vi "Read Full Output.vi"(6 "maximal byte count (-1)":i32=-1, 7 "timeout [ms]":u32, 8 "error in":errorcluster, 11 "GOLPI ref. in":T1={"pipe handle"={"lv_proc.dll file path"=path "", "process instance handle"=[], "debug mode"=FALSE, "debug data"=[]}, "fast read timeout [ms]"=500, "fast read settle time [ms]"=10, "fast read to multiple [ms]"=1, "max elements per input line"=100, "slow read timeout [ms]"=5000, "stdin double format specifier"="%_16e", "max elements per stdout output column"=100}) -> (0 "error out":errorcluster, 2 "read buffer":string, 3 "GOLPI ref. out":T1={"pipe handle"={"lv_proc.dll file path"=path "", "process instance handle"=[], "debug mode"=FALSE, "debug data"=[]}, "fast read timeout [ms]"=500, "fast read settle time [ms]"=10, "fast read to multiple [ms]"=1, "max elements per input line"=100, "slow read timeout [ms]"=5000, "stdin double format specifier"="%_16e", "max elements per stdout output column"=100}, 5 "bytes remaining":i32)   [LabVIEW 2013, in "GOLPI library.lvlib"]
doc: "Reads full output of GNU Octave in stdout pipe.\nIf timeout is exceeded (i.e. buffer contains too many characters), returns only part of buffer and returns number of bytes remaining in the stdout (if any).\nReading also stops if maximal byte count terminal is set to natural nonzero value and number of red bytes reaches this limit."
uses:
  GOLPI library.lvlib
  Private/Type Definitions/GOLPI reference Type Def.ctl
  LV Process source distribution/Pipe Handle.ctl
  Private/Type Definitions/Custom Error Codes Enum Type Def.vi
  LV Process source distribution/LV Process library.lvlib
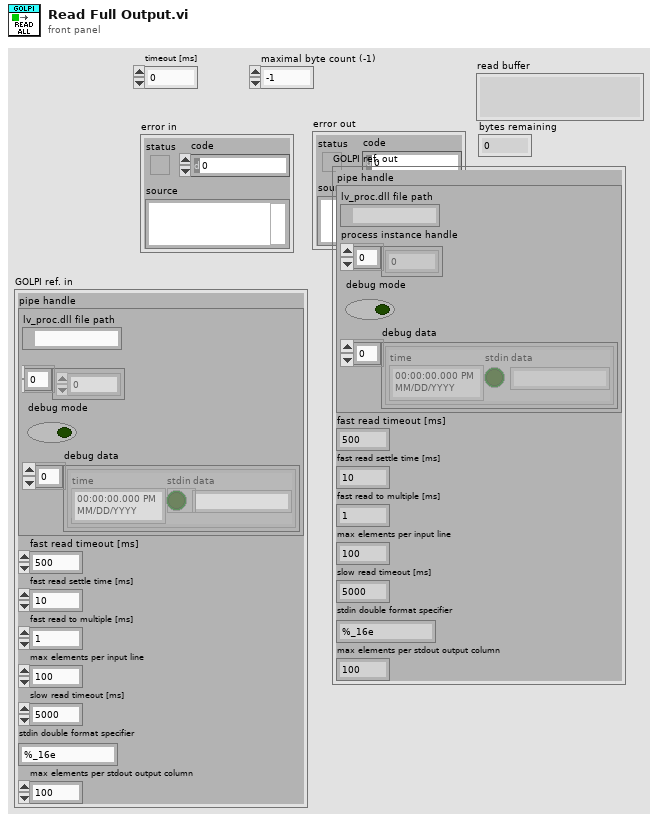
[diagram p1: front panel]
types:
  T1 = typedef "GOLPI library.lvlib/GOLPI reference Type Def.ctl" = cluster{"pipe handle":T2, "fast read timeout [ms]":u32, "fast read settle time [ms]":u32, "fast read to multiple [ms]":u32, "max elements per input line":u32, "slow read timeout [ms]":u32, "stdin double format specifier":string, "max elements per stdout output column":u32}
  T2 = typedef "LV Process library.lvlib/Pipe Handle.ctl" = cluster{"lv_proc.dll file path":path, "process instance handle":u32[], "debug mode":bool, "debug data":cluster{"time":timestamp, "stdin":bool, "data":string}[]}
  T3 = typedef "GOLPI library.lvlib/Custom Error Codes Enum Type Def.vi" = enum16{"no error", "00 working directory PAR1 missing", "01 octave binary PAR1 missing", "02 octave report error PAR1", "03 empty output last cmd PAR1", "04 missing temporary file PAR1", "05 pwd PAR 1 not exist", "10 var PAR1 not string, vect", "11 var PAR1 not num, scal, ~compl", "12 var PAR1 not num, scal, compl", "13 var PAR1 not num, vect, ~compl", "14 var PAR1 not num, vect, compl", "15 var PAR1 not num, mat, ~compl", "16 var PAR1 not num, mat, ~compl", "30 WARNING read timeout", "99 not finished"}
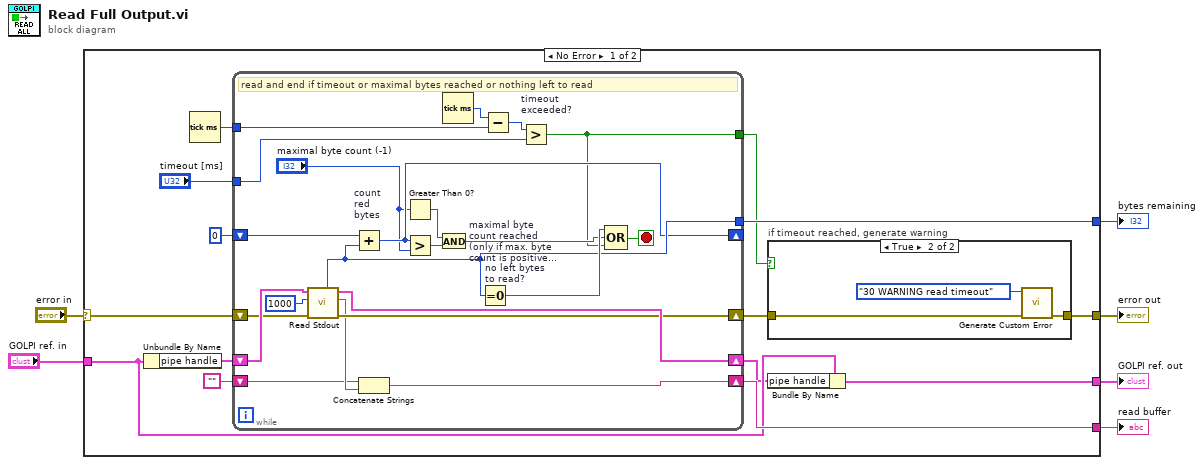
[diagram p0: block diagram]
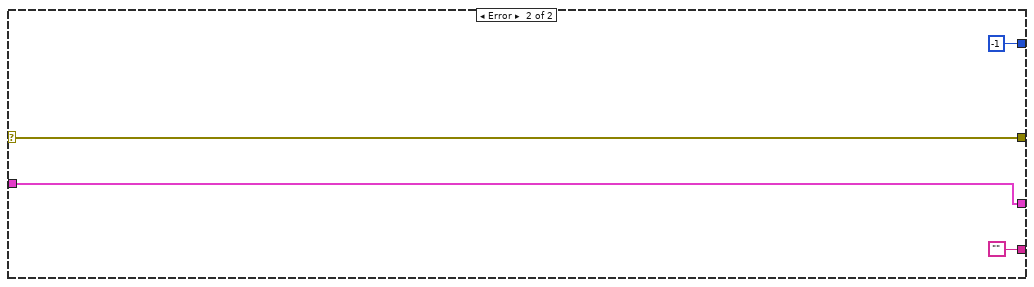
[diagram p3: hidden frame]
diagram:
  n1 = case shown="No Error" "error in" {
    selector: "error in" -> [w7 w47]
    tunnel: [w20 ""] -> w6
    tunnel: [w19 -1 ("bytes remaining")] -> w5
    tunnel: "GOLPI ref. in" -> [w14 w50]
    tunnel: [w13 w50] -> w3
    tunnel: [w10 w47] -> w2
    frame No Error {
      n2 = Unbundle By Name(w14) -> ("pipe handle"=w12:T2)
      n3 = Tick Count (ms)() -> (millisecond timer value=w17:u32)
      n4 = while {
        tunnel: [w31] -> w19
        shift-right: [w45] -> w11
        shift-left: w12 -> [w46]
        shift-right: [w40] -> w20
        shift-left: "" -> [w41]
        tunnel: w17 -> [w38]
        tunnel: "timeout [ms]" -> [w35]
        shift-right: [w30] -> _
        shift-left: 0 -> [w33]
        shift-right: [w44] -> w9
        shift-left: w7 -> [w43]
        tunnel: [w25] -> w8
        stop <- w34 stop-if-true
        # "read and end if timeout or maximal bytes reached or nothing left to read"
        n5 = call "Read Stdout.vi"("error in"=w43, "byte count"=1000, "pipe in"=w46) -> ("error out"=w44:errorcluster, "read buffer"=w42:string, "pipe out"=w45:T2, "bytes remaining"=w31:i32)  [unwired: 3 in, 2 out]
        n6 = Add "count\nred\nbytes"(x=w33, y=w31) -> (x+y=w30:i32)
        n7 = Concatenate Strings(w41, w42) -> (w40:string)
        n8 = Greater Than 0?(x="maximal byte count (-1)") -> (x > 0?=w29:bool)
        n9 = Greater?(x=w30, y="maximal byte count (-1)") -> (0:w27:bool)
        n10 = And "maximal byte\ncount reached\n(only if max. byte\ncount is positive\nand nonzero)?"(x=w29, y=w27) -> (x .and. y?=w26:bool)
        n11 = Tick Count (ms)() -> (millisecond timer value=w39:u32)
        n12 = Equal To 0? "no left bytes\nto read?"(x=w31) -> (x = 0?=w36:bool)
        n13 = Subtract(x=w39, y=w38) -> (x-y=w37:u32)
        n14 = Greater? "timeout\nexceeded?"(x=w37, y=w35) -> (0:w25:bool)
        n15 = Compound Arithmetic op=OR(w36, w26, w25) -> (w34:bool)
      }
      n16 = case "if timeout reached, generate warning" shown="True" w8 {
        tunnel: [w21 w22] -> w10
        tunnel: w9 -> [w21 w23]
        frame False {
        }
        frame True {
          n17 = call "Generate Custom Error.vi"("error in"=w23, "GOLPI error"=Custom_Error_Codes_Enum_Type_Def.vi."30 WARNING read timeout") -> ("error out"=w22:errorcluster)  [unwired: 9 in]
        }
      }
      n18 = Bundle By Name(cluster=w14, "pipe handle"=w11) -> (w13:T1)
    }
    frame Error {
    }
  }
  "error out" <- w2
  "read buffer" <- w6
  "bytes remaining" <- w5
  "GOLPI ref. out" <- w3
